vi "Then.vi"(7 "Then Promise":refnum<class "Promise.lvclass">, 10 "error in (no error)":errorcluster, 11 "Future in":refnum<class "Future.lvclass">) -> (2 "error out":errorcluster, 3 "Future out":refnum<class "Future.lvclass">)   [LabVIEW 2020, in "Promises.lvlib" / "Future.lvclass"]
doc: "Chains additional futures for futher work based on the successful result, handling errors, and work regardless of success or failure."
uses:
  Future.lvclass
  Promise/Promise.lvclass
  Future.lvclass/Future.ctl
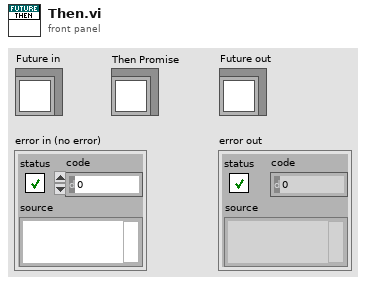
[diagram p1: front panel]
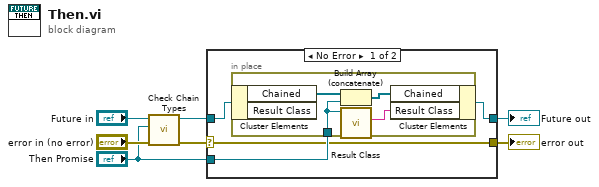
[diagram p0: block diagram]
diagram:
  n1 = call "Check Chain Types.vi"("error in (no error)"="error in (no error)", "Then"="Then Promise", "Future in"="Future in") -> ("error out"=w3:errorcluster, "Future out"=w4:refnum<class "Future.lvclass">)  [unwired: 7 in]
  n2 = case shown="No Error" w3 {
    selector: w3 -> [w8 w16]
    tunnel: [w9 w17] -> w6
    tunnel: w4 -> [w11 w17]
    tunnel: "Then Promise" -> [w10 _]
    tunnel: [w8 w16] -> w2
    frame No Error {
      n3 = in-place {
        in-place-border: w10 -> [w13]
        n4 = in-place-cluster #1(w11) -> ("Chained"=w15:refnum<class "Promise.lvclass">[])  [unwired: 1 out]
        n5 = Build Array (concatenate)(w15, w13) -> (w12:refnum<class "Promise.lvclass">[])
        n6 = call "Result Class.vi"("Promise in"=w13) -> ("Result Class"=w14:string)  [unwired: 10 in]
        n7 = in-place-cluster #1("Chained"=w12, "Result Class"=w14) -> (w9:refnum<class "Future.lvclass">)
      }
    }
    frame Error {
    }
  }
  "error out" <- w2
  "Future out" <- w6
